vi "VG_branche.vi"() -> ()   [LabVIEW 2020]
panel:
  out "Branche":dbl=1.0
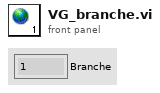
[diagram p1: front panel]
diagram:
